vi "Update Actor Attributes.vi"(7 "Actor in":refnum<class "Actor.lvclass">, 10 "This VI":refnum<vi>) -> (0 "Error out":errorcluster, 5 "Actor out":refnum<class "Actor.lvclass">)   [LabVIEW 2020, in "jettl.lvlib"]
uses:
  jettl.lvlib
  Msg/Msg.lvclass
  Actor/Actor.lvclass
  Msg Input/Msg Input.lvclass
  Msg Output/Msg Output.lvclass
  Unified Actor Relation.ctl
  Teller.ctl
  Msg.ctl
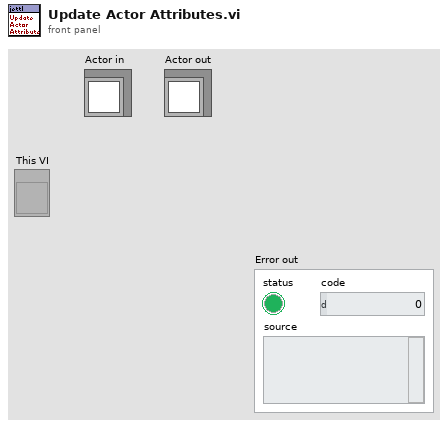
[diagram p1: front panel]
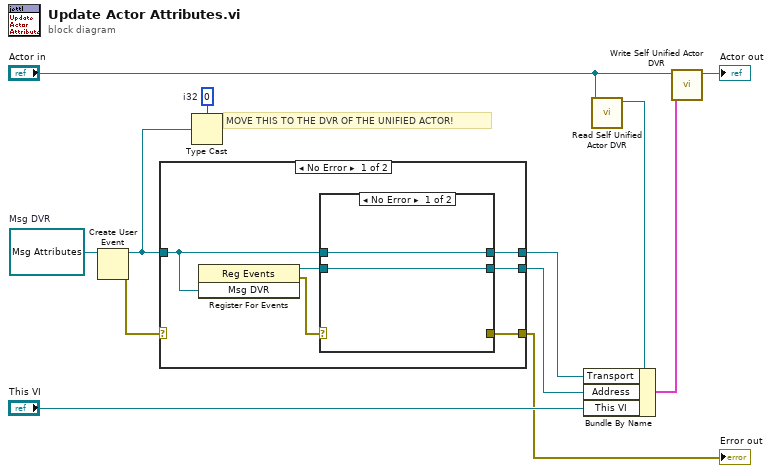
[diagram p0: block diagram]
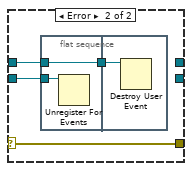
[diagram p2: hidden frame]
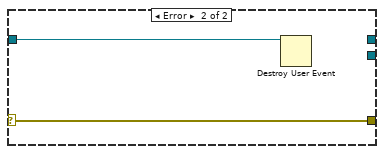
[diagram p3: hidden frame]
diagram:
  w3 = refnum<data-value> refnum  # Msg DVR
  w7 = 0  # i32
  # "MOVE THIS TO THE DVR OF THE UNIFIED ACTOR!"
  n1 = Create User Event(user event datatype=w3) -> (user event=w8:refnum<user-event>, error out=w9:errorcluster)  [unwired: 1 in]
  n2 = case shown="No Error" w9 {
    selector: w9 -> [_ w29]
    tunnel: [w18 w29] -> w6
    tunnel: w8 -> [w13 w28]
    tunnel: [w17 _] -> w2
    tunnel: [w16 _] -> w1
    frame No Error {
      n3 = register-events(w13) -> (reference out=w14:refnum<event-registration>, error out=w15:errorcluster)  [unwired: 2 in]
      n4 = case shown="No Error" w15 {
        selector: w15 -> [_ w24]
        tunnel: [_ w24] -> w18
        tunnel: [w20 _] -> w16
        tunnel: w14 -> [w20 w23]
        tunnel: [w19 _] -> w17
        tunnel: w13 -> [w19 w21]
        frame No Error {
        }
        frame Error {
          n5 = flat-sequence {
            tunnel: w23 -> [w26]
            tunnel: [w25] -> w22
            tunnel: w21 -> [w25]
            tunnel: w22 -> [w27]
            frame #0 {
              n6 = Unregister For Events(event registration refnum=w26) -> ()  [unwired: 1 in, 1 out]
            }
            frame #1 {
              n7 = Destroy User Event(user event=w27) -> ()  [unwired: 1 in, 1 out]
            }
          }
        }
      }
    }
    frame Error {
      n8 = Destroy User Event(user event=w28) -> ()  [unwired: 1 in, 1 out]
    }
  }
  "Error out" <- w6
  n9 = Type Cast(type=w7, x=w8) -> ()  [unwired: 1 out]
  n10 = call-dynamic "Read Self Unified Actor DVR.vi"("Actor in"="Actor in") -> ("Self Unified Actor DVR"=w5:refnum<data-value>)  [unwired: 10 in]
  n11 = Bundle By Name(cluster=w5, "Transport"=w2, "Address"=w1, "This VI"="This VI") -> (w4:cluster{})
  n12 = call-dynamic "Write Self Unified Actor DVR.vi"("Self Unified Actor DVR"=w4, "Actor in"="Actor in") -> ("Actor out"=→"Actor out":refnum<class "Actor.lvclass">)  [unwired: 9 in]
